vi "Convert Image To Base64.vi"(8 "error in (no error)":errorcluster, 11 "Get Control Value Variant":variant) -> (0 "error out":errorcluster, 3 "<JSON>":string)   [LabVIEW 2025, in "MCP Server.lvlib"]
uses:
  MCP Server.lvlib
  <vilib>/Utility/sysdir.llb/System Directory Type.ctl
  <vilib>/JDP Science/JDP Science Common Utilities/Base64/Base64 Support.lvlib
panel:
  out "new picture":picture
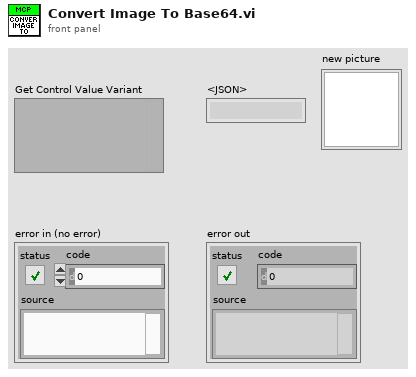
[diagram p1: front panel]
types:
  T1 = typedef "imagedata.ctl" = cluster{"image type":i32, "image depth":i32, "image":u8[], "mask":u8[], "colors":u32[], "Rectangle":cluster{"left":i16, "top":i16, "right":i16, "bottom":i16}}
  T2 = typedef "System Directory Type.ctl" = i32
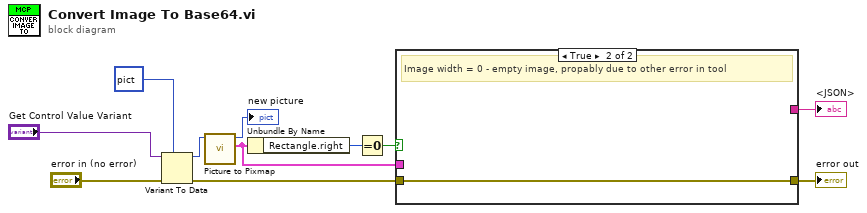
[diagram p0: block diagram]
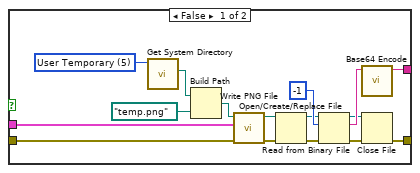
[diagram p2: hidden frame]
diagram:
  n1 = Variant To Data(error in="error in (no error)", type=picture data[5B] ("picture"), Variant="Get Control Value Variant") -> (data=w8:picture, error out=w5:errorcluster)
  n2 = call <vilib>:"Picture to Pixmap.vi"("picture"=w8) -> ("image data"=w3:T1, "new picture"=→"new picture":picture)  [unwired: 9 in]
  n3 = Unbundle By Name(w3) -> ("Rectangle.right"=w2:i16)
  n4 = Equal To 0?(x=w2) -> (x = 0?=w1:bool)
  n5 = case shown="True" w1 {
    tunnel: [w16 w28] -> w6
    tunnel: w5 -> [w14 w28]
    tunnel: [w13 _] -> w4
    tunnel: w3 -> [w12 _]
    frame False {
      w18 = T2 5 items=["User Home"=0, "User Desktop"=1, "User Documents"=2, "User Application Data"=3, "User Preferences"=4, "User Temporary"=5, "Public Documents"=6, "Public Application Data"=7, "Public Preferences"=8, "Public Cache"=13, "System Core Libraries"=9, "System Installed Libraries"=10, "Application Files"=11, "Boot Volume Root"=12] ("system directory type")
      n6 = call <vilib>:"Get System Directory.vi"("system directory type"=w18) -> ("system directory"=w19:path)  [unwired: 10 in]
      n7 = Build Path(base path=w19, name or relative path=path "temp.png") -> (appended path=w20:path)
      n8 = call <vilib>:"Write PNG File.vi"("error in (no error)"=w14, "image data"=w12, "path to PNG file"=w20) -> ("error out"=w15:errorcluster, "path"=w17:path)  [unwired: 7 in]
      n9 = Open/Create/Replace File(file path (use dialog)=w17, error in=w15) -> (refnum out=w25:refnum<file>, error out=w22:errorcluster)  [unwired: 4 in, 1 out]
      n10 = Read from Binary File(8:w22, 10:-1 ("count (1)"), 11:w25) -> (0:w23:errorcluster, 2:w26:string, 3:w24:refnum<file>)  [unwired: 3 in, 1 out]
      n11 = call <vilib>:"Base64 Encode.vi"("String to Encode"=w26) -> ("Base64 Encoded"=w13:string)  [unwired: 10 in]
      n12 = Close File(refnum=w24, error in=w23) -> (error out=w16:errorcluster)  [unwired: 1 out]
    }
    frame True {
      # "Image width = 0 - empty image, propably due to other error in tool"
    }
  }
  "error out" <- w6
  "<JSON>" <- w4
